vi "ErrorHandling.loadPastErrors.vi"(8 "error in (no error)":errorcluster, 11 "ErrorHandling in":refnum<data-value>) -> (0 "error out":errorcluster, 3 "ErrorHandling out":refnum<data-value>)   [LabVIEW 2016, in "ErrorHandling.lvclass"]
doc: "Lädt den Inhalt der Error-Log Datei\n\n27.05.14 / sige"
uses:
  ErrorHandling.lvclass
  ErrorHandling.lvclass/ErrorHandling.ctl
  ErrorHandling.OccurredErrorDataStruct.ctl
  <vilib>/Utility/error.llb/Search and Replace Pattern.vi
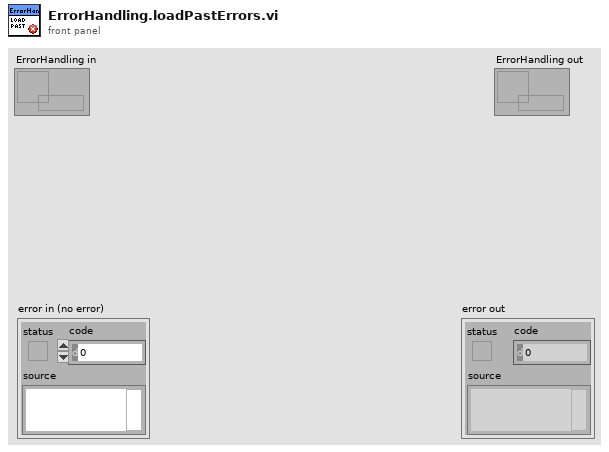
[diagram p1: front panel]
types:
  T1 = enum16{"open", "replace", "create", "open or create", "replace or create", "replace or create with confirmation"}
  T2 = typedef "ErrorHandling.lvclass/ErrorHandling.OccurredErrorDataStruct.ctl" = cluster{"Error":errorcluster, "Caller":string, "Comment":string, "Timestamp":timestamp, "Stopped":bool, "ErrorCusterString":string, "ErrorIndex":u64}
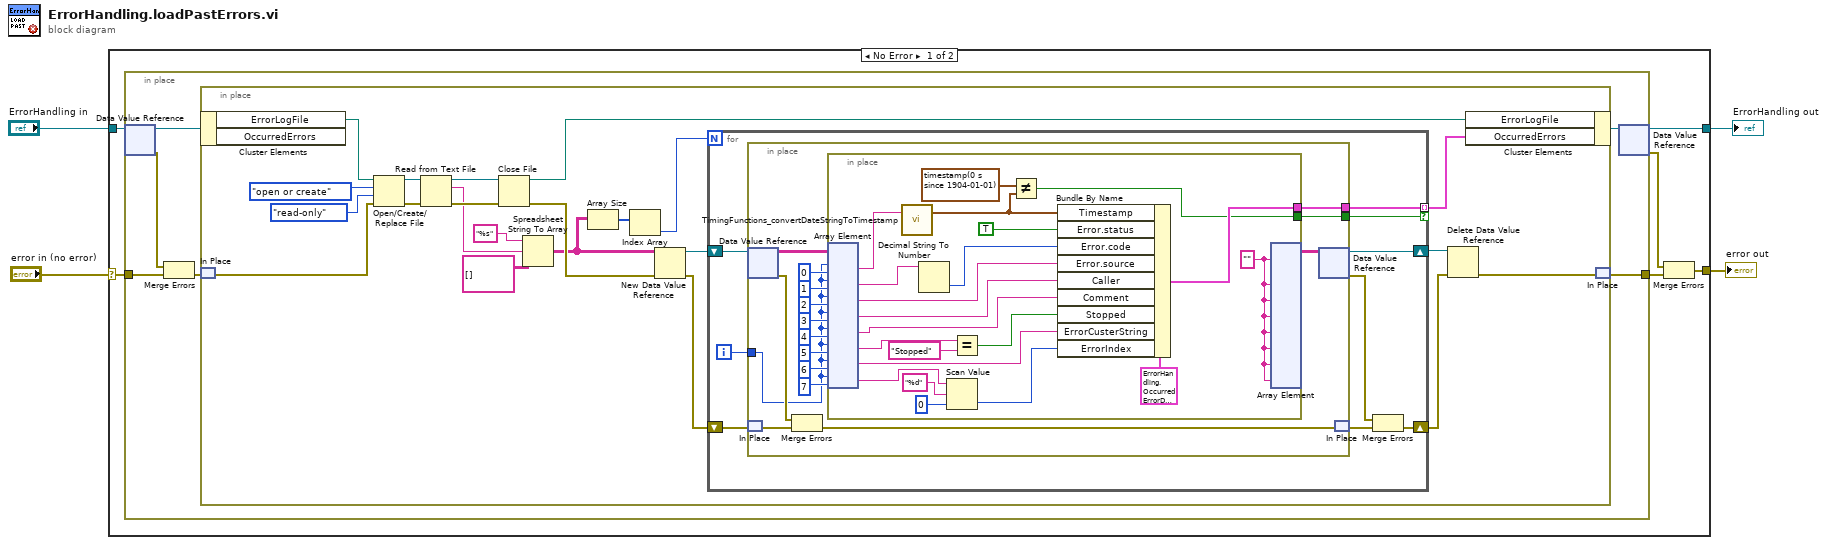
[diagram p0: block diagram]
diagram:
  n1 = case shown="No Error" "error in (no error)" {
    selector: "error in (no error)" -> [w10 w86]
    tunnel: [w5 w86] -> w3
    tunnel: "ErrorHandling in" -> [w9 w85]
    tunnel: [w8 w85] -> w1
    frame No Error {
      n2 = in-place {
        in-place-border: w10 -> [w13]
        in-place-border: [w16] -> w6
        n3 = in-place-dvr #1(w9) -> (w15:refnum<class "ErrorHandling.lvclass">, w12:errorcluster)
        n4 = Merge Errors(w12, w13) -> (w11:errorcluster)
        n5 = in-place {
          n6 = in-place-cluster #2(w15) -> ("ErrorLogFile"=w27:path)  [unwired: 1 out]
          n7 = in-place-match #3(w11) -> (w28:errorcluster)
          n8 = Open/Create/Replace File(file path (use dialog)=w27, error in=w28, operation (0:open)=T1."open or create", access (0:read/write)=enum16{"read/write", "read-only", "write-only"}."read-only") -> (refnum out=w34:refnum<file>, error out=w33:errorcluster)  [unwired: 2 in, 1 out]
          n9 = Read from Text File(file (use dialog)=w34, error in=w33) -> (refnum out=w36:refnum<file>, text=w31:string, error out=w35:errorcluster)  [unwired: 2 in, 1 out]
          n10 = Close File(refnum=w36, error in=w35) -> (path=w26:path, error out=w38:errorcluster)
          n11 = Spreadsheet String To Array(format string="%s", spreadsheet string=w31, array type (2D Dbl)=string[][] []) -> (array=w23:string[][])  [unwired: 1 in]
          n12 = Array Size(array=w23) -> (size(s)=w22:i32[])
          n13 = Index Array(array=w22) -> (element=w21:i32)  [unwired: 1 in]
          n14 = New Data Value Reference(data value=w23, error in=w38) -> (data value reference=w24:refnum<data-value>, error out=w18:errorcluster)
          n15 = for {
            N: w21 -> [_]
            tunnel: [w47] -> w25 mode=indexing if=w46
            shift-right: [w43] -> w20
            shift-left: w24 -> [w45]
            shift-right: [w40] -> w19
            shift-left: w18 -> [w39]
            i -> [w44]
            n16 = in-place {
              in-place-border: [w63] -> w47
              in-place-border: [w62] -> w46
              in-place-border: w44 -> [w48]
              n17 = in-place-dvr #4(w45) -> (w61:string[][], w59:errorcluster)
              n18 = in-place-match #5(w39) -> (w57:errorcluster)
              n19 = Merge Errors(w59, w57) -> (w58:errorcluster)
              n20 = in-place {
                in-place-border: [w81] -> w63
                in-place-border: [w78] -> w62
                w65 = "" ("element")
                n21 = in-place-array #6(w61, w48, 0, w48, 1, w48, 2, w48, 3, w48, 4, w48, 5, w48, 6, w48, 7) -> (w73:string, w72:string, w71:string, w70:string, w66:string, w67:string, w68:string, w69:string)
                n22 = call "TimingFunctions_convertDateStringToTimestamp.vi"("TimeStamp (yymmdd HHMMSS)"=w73) -> ("TimeStamp (LV)"=w80:timestamp)  [unwired: 17 in, 1 out]
                n23 = Decimal String To Number(string=w72) -> (number=w83:i32)  [unwired: 2 in, 1 out]
                n24 = Scan Value(string=w69, format string="%d", default (0 dbl)=u64 0) -> (value=w75:u64)  [unwired: 1 out]
                n25 = Equal?(x=w67, y="Stopped") -> (x = y?=w77:bool)
                n26 = Not Equal?(x=timestamp(0 s since 1904-01-01), y=w80) -> (x != y?=w78:bool)
                n27 = Bundle By Name(cluster=T2 {"Error"={"status"=FALSE, "code"=0, "source"=""}, "Caller"="", "Comment"="", "Timestamp"=timestamp(0 s since 1904-01-01), "Stopped"=FALSE, "ErrorCusterString"="", "ErrorIndex"=0} ("Cluster"), "Timestamp"=w80, "Error.status"=TRUE, "Error.code"=w83, "Error.source"=w71, "Caller"=w70, "Comment"=w66, "Stopped"=w77, "ErrorCusterString"=w68, "ErrorIndex"=w75) -> (w81:T2)
                n28 = in-place-array #6(w65, w65, w65, w65, w65, w65, w65, w65) -> (w60:string[][])  [unwired: 16 out]
              }
              n29 = in-place-dvr #4(w60) -> (w43:refnum<data-value>, w42:errorcluster)
              n30 = in-place-match #5(w58) -> (w41:errorcluster)
            }
            n31 = Merge Errors(w42, w41) -> (w40:errorcluster)
          }
          n32 = Delete Data Value Reference(data value reference=w20, error in=w19) -> (error out=w17:errorcluster)  [unwired: 1 out]
          n33 = in-place-cluster #2("ErrorLogFile"=w26, "OccurredErrors"=w25) -> (w14:refnum<class "ErrorHandling.lvclass">)
          n34 = in-place-match #3(w17) -> (w16:errorcluster)
        }
        n35 = in-place-dvr #1(w14) -> (w8:refnum<data-value>, w7:errorcluster)
      }
      n36 = Merge Errors(w7, w6) -> (w5:errorcluster)
    }
    frame Error {
    }
  }
  "error out" <- w3
  "ErrorHandling out" <- w1
